vi "mobileye_decoder.vi"(10 "can cluster":T1 {"identifier" format="%03x"}, 11 "name":string="Mobileye560") -> ()   [LabVIEW 2015]
uses:
  rio_Global.vi
panel:
  out "next lane right":dbl[][](array[numeric])
  out "next lane left":dbl[][](array[numeric])
  out "lane_right":dbl[](array[numeric])
  out "lane_left":dbl[](array[numeric])
  out "obs_tmp":dbl[][](array[numeric])
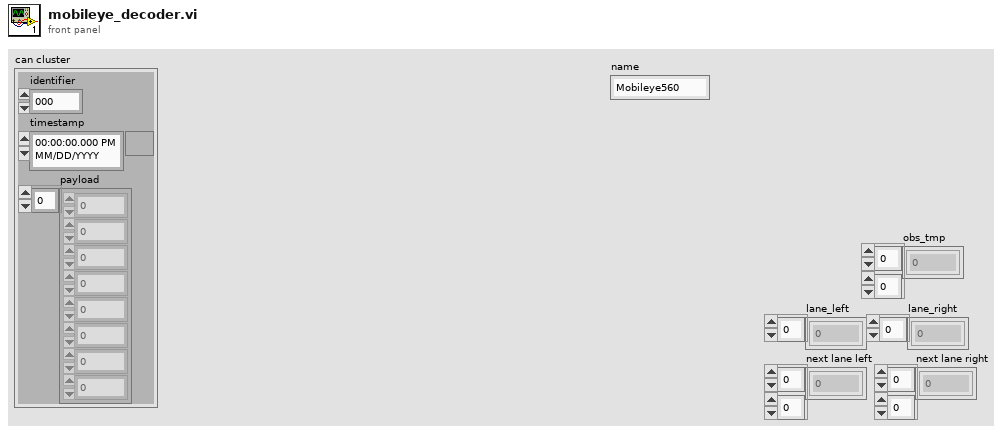
[diagram p1: front panel]
types:
  T1 = cluster{"identifier":u32, "timestamp":timestamp, "payload":u8[]}
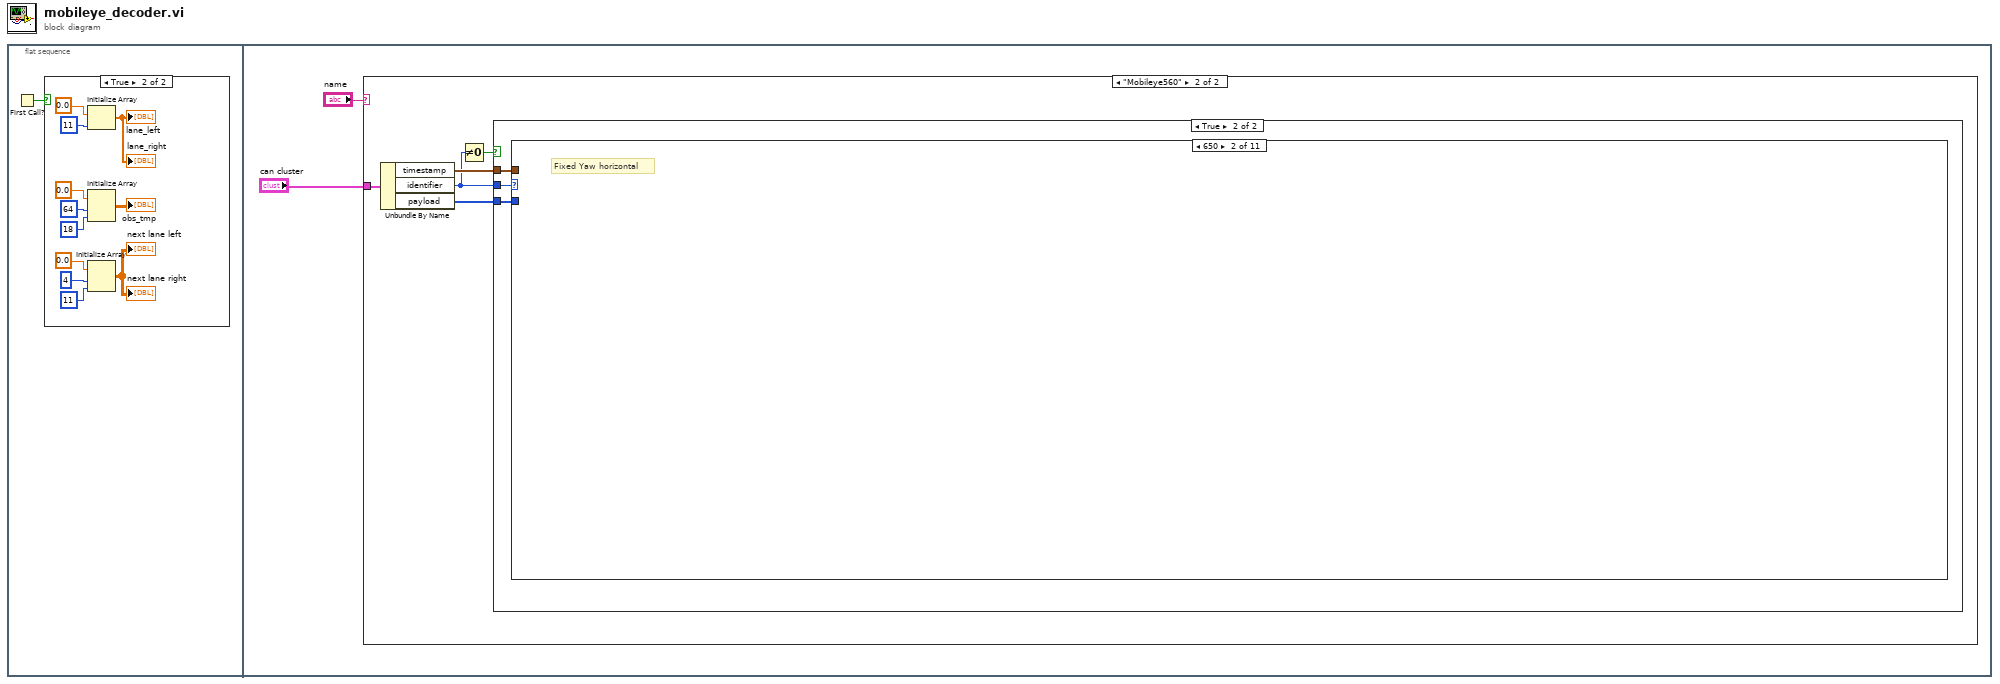
[diagram p0: block diagram]
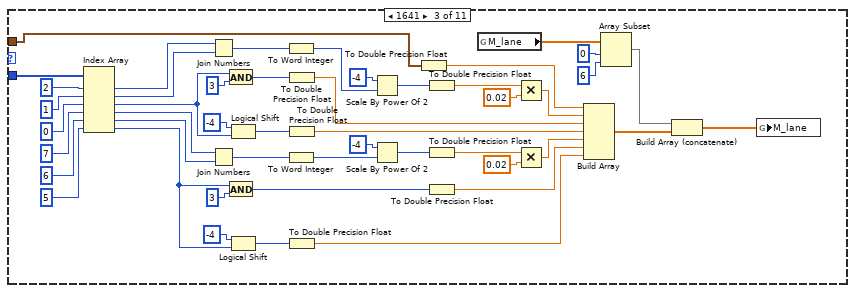
[diagram p6: hidden frame]
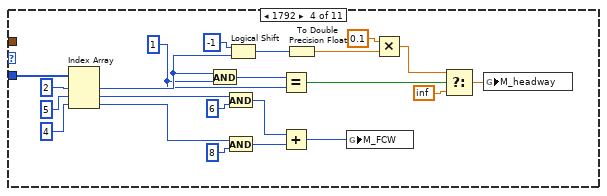
[diagram p7: hidden frame]
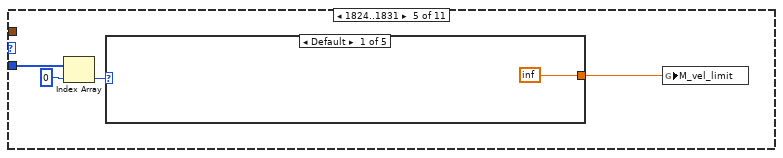
[diagram p8: hidden frame]
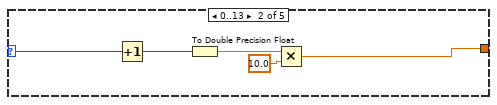
[diagram p9: hidden frame]
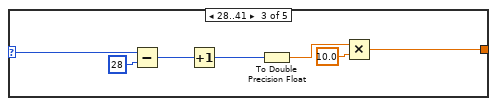
[diagram p10: hidden frame]
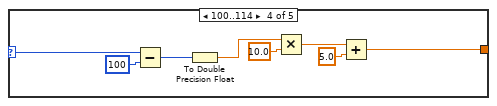
[diagram p11: hidden frame]
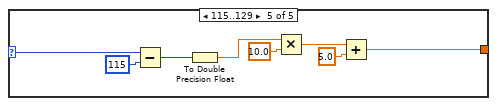
[diagram p12: hidden frame]
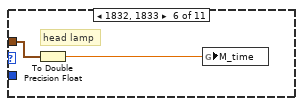
[diagram p13: hidden frame]
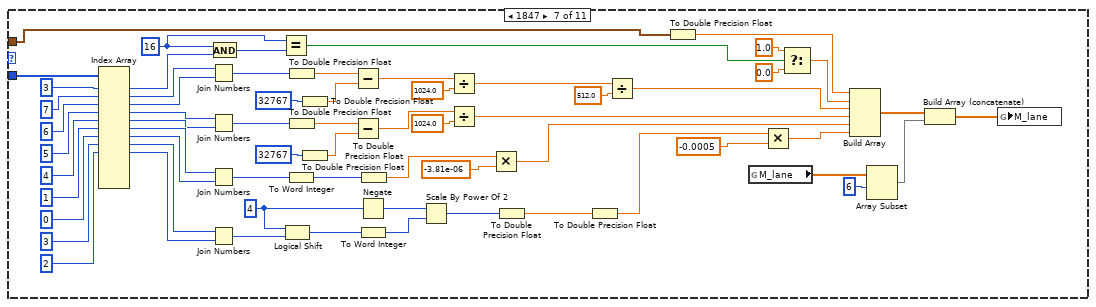
[diagram p14: hidden frame]
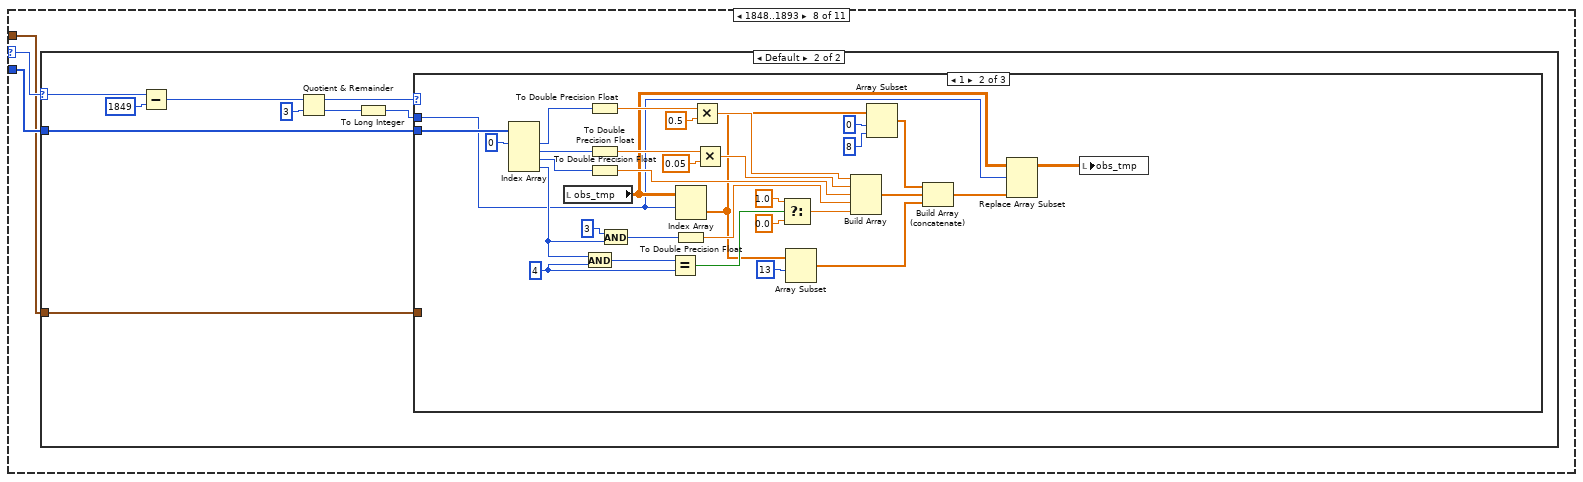
[diagram p15: hidden frame]
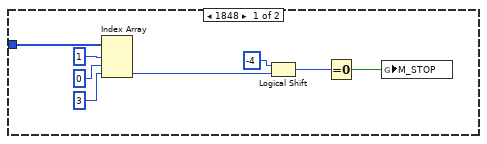
[diagram p16: hidden frame]
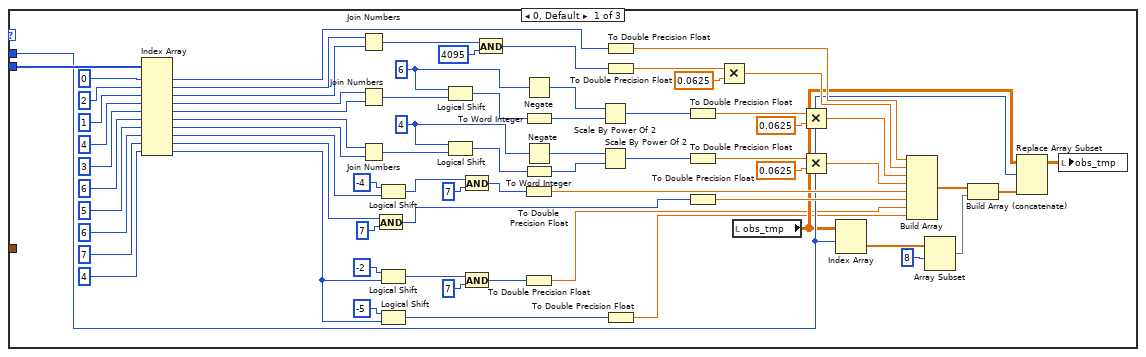
[diagram p17: hidden frame]
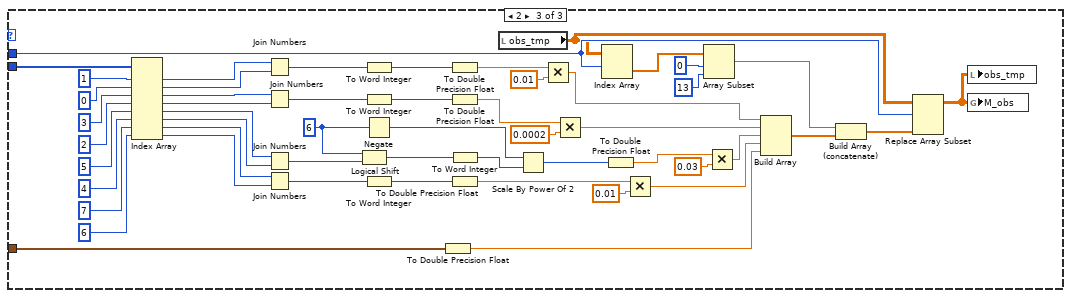
[diagram p18: hidden frame]
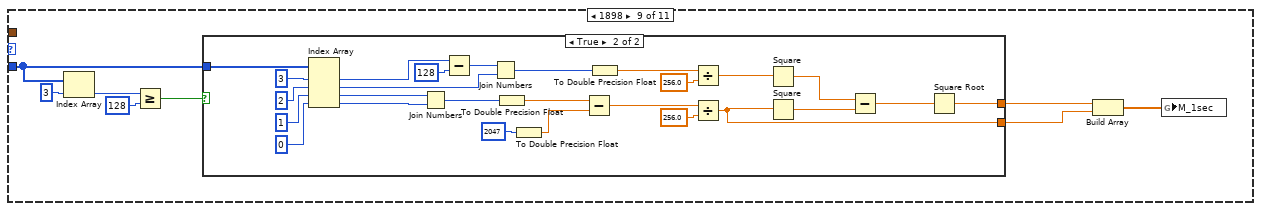
[diagram p19: hidden frame]
diagram:
  n1 = flat-sequence {
    frame #0 {
      n2 = First Call?() -> (First Call?: T/F=w1:bool)
      n3 = case shown="True" w1 {
        frame False {
        }
        frame True {
          n4 = Initialize Array(0.0, 11 ("dimension size")) -> (→"lane_left" →"lane_right":dbl[])
          n5 = Initialize Array(0.0 ("element"), 64 ("dimension size"), 18 ("dimension size")) -> (→"obs_tmp":dbl[][])
          n6 = Initialize Array(0.0, 4 ("dimension size"), 11 ("dimension size")) -> (→"next lane left" →"next lane right":dbl[][])
        }
      }
    }
    frame #1 {
      n7 = case shown="\"Mobileye560\"" "name" {
        tunnel: "can cluster" -> [_ w19]
        frame "False", Default {
        }
        frame "Mobileye560" {
          n8 = Unbundle By Name(w19) -> ("timestamp"=w17:timestamp, "identifier"=w16:u32, "payload"=w18:u8[])
          n9 = Not Equal To 0?(x=w16) -> (x != 0?=w15:bool)
          n10 = case shown="True" w15 {
            tunnel: w18 -> [_ w22]
            tunnel: w17 -> [_ w21]
            tunnel: w16 -> [_ w20]
            frame False {
            }
            frame True {
              n11 = case shown="650" w20 {
                selector: w20 -> [_ _ _ _ _ _ _ w192 _ w399 w480]
                tunnel: w22 -> [_ _ w69 w91 w95 _ w189 w191 w368 w453 w508]
                tunnel: w21 -> [_ _ w46 _ _ w126 w133 w190 _ w419 w483]
                frame 0, Default {
                }
                frame 1616 {
                  # "Fixed Yaw horizontal"
                }
                frame 1641 {
                  n12 = Index Array(array=w69, index #1=2 ("index"), index #2=1 ("index"), index #3=0 ("index"), index #4=7 ("index"), index #5=6 ("index"), index #6=5 ("index")) -> (element #1=w66:u8, element #2=w65:u8, element #3=w44:u8, element #4=w37:u8, element #5=w36:u8, element #6=w32:u8)
                  n13 = Join Numbers(hi=w66, lo=w65) -> ((hi.lo)=w64:u16)
                  n14 = Join Numbers(hi=w37, lo=w36) -> ((hi.lo)=w59:u16)
                  n15 = And(x=w44, y=u8 3) -> (x .and. y?=w43:u8)
                  n16 = And(x=w32, y=u8 3) -> (x .and. y?=w35:u8)
                  n17 = Logical Shift(y=i16 -4, x=w44) -> (x << y=w42:u8)
                  n18 = Logical Shift(y=i16 -4, x=w32) -> (x << y=w39:u8)
                  n19 = To Word Integer(number=w64) -> (16bit integer=w51:i16)
                  n20 = To Word Integer(number=w59) -> (16bit integer=w48:i16)
                  n21 = To Double Precision Float(number=w43) -> (double precision float=w41:dbl)
                  n22 = To Double Precision Float(number=w42) -> (double precision float=w40:dbl)
                  n23 = To Double Precision Float(number=w39) -> (double precision float=w33:dbl)
                  n24 = Scale By Power Of 2(n=i16 -4 ("y"), x=w51) -> (x*2^n=w50:i16)
                  n25 = Scale By Power Of 2(n=i16 -4 ("y"), x=w48) -> (x*2^n=w47:i16)
                  n26 = To Double Precision Float(number=w46) -> (double precision float=w31:dbl)
                  n27 = To Double Precision Float(number=w50) -> (double precision float=w63:dbl)
                  n28 = To Double Precision Float(number=w47) -> (double precision float=w60:dbl)
                  n29 = To Double Precision Float(number=w35) -> (double precision float=w34:dbl)
                  n30 = global read "rio_Global.vi" "M_lane"() -> (w23:dbl[])
                  n31 = Multiply(x=w63, y=0.02) -> (x*y=w26:dbl)
                  n32 = Multiply(x=w60, y=0.02) -> (x*y=w25:dbl)
                  n33 = Build Array(w31, w26, w41, w40, w25, w34, w33) -> (w27:dbl[])
                  n34 = Array Subset(array=w23, index=0, length=6) -> (w28:dbl[])
                  n35 = Build Array (concatenate)(w28, w27) -> (w24:dbl[])
                  n36 = global write "rio_Global.vi" "M_lane"(w24) -> ()
                }
                frame 1792 {
                  w86 = u8 1 ("y")
                  n37 = Index Array(array=w91, index #1=2 ("index"), index #2=5 ("index"), index #3=4 ("index")) -> (element #1=w89:u8, element #2=w78:u8, element #3=w74:u8)
                  n38 = And(x=w89, y=w86) -> (x .and. y?=w87:u8)
                  n39 = And(x=w78, y=u8 6) -> (x .and. y?=w73:u8)
                  n40 = And(x=w74, y=u8 8) -> (x .and. y?=w72:u8)
                  n41 = Logical Shift(y=i16 -1, x=w89) -> (x << y=w84:u8)
                  n42 = Equal?(x=w87, y=w86) -> (x = y?=w85:bool)
                  n43 = Add(x=w73, y=w72) -> (x+y=w70:u8)
                  n44 = To Double Precision Float(number=w84) -> (double precision float=w83:dbl)
                  n45 = global write "rio_Global.vi" "M_FCW"(w70) -> ()
                  n46 = Multiply(x=0.1, y=w83) -> (x*y=w81:dbl)
                  n47 = Select(t=w81, s=w85, f=inf) -> (s? t:f=w71:dbl)
                  n48 = global write "rio_Global.vi" "M_headway"(w71) -> ()
                }
                frame 1824..1831 {
                  n49 = Index Array(array=w95, index=0) -> (element=w93:u8)
                  n50 = case shown="Default" w93 {
                    selector: w93 -> [_ w101 w104 w114 w122]
                    tunnel: [inf w97 w105 w109 w117] -> w92
                    frame Default {
                    }
                    frame 0..13 {
                      n51 = Increment(x=w101) -> (x+1=w100:u8)
                      n52 = To Double Precision Float(number=w100) -> (double precision float=w99:dbl)
                      n53 = Multiply(x=w99, y=10.0) -> (x*y=w97:dbl)
                    }
                    frame 28..41 {
                      n54 = Subtract(x=w104, y=u8 28) -> (x-y=w103:u8)
                      n55 = Increment(x=w103) -> (x+1=w108:u8)
                      n56 = To Double Precision Float(number=w108) -> (double precision float=w107:dbl)
                      n57 = Multiply(x=w107, y=10.0) -> (x*y=w105:dbl)
                    }
                    frame 100..114 {
                      n58 = Subtract(x=w114, y=u8 100) -> (x-y=w112:u8)
                      n59 = To Double Precision Float(number=w112) -> (double precision float=w116:dbl)
                      n60 = Multiply(x=w116, y=10.0) -> (x*y=w111:dbl)
                      n61 = Add(x=w111, y=5.0) -> (x+y=w109:dbl)
                    }
                    frame 115..129 {
                      n62 = Subtract(x=w122, y=u8 115) -> (x-y=w120:u8)
                      n63 = To Double Precision Float(number=w120) -> (double precision float=w124:dbl)
                      n64 = Multiply(x=w124, y=10.0) -> (x*y=w119:dbl)
                      n65 = Add(x=w119, y=5.0) -> (x+y=w117:dbl)
                    }
                  }
                  n66 = global write "rio_Global.vi" "M_vel_limit"(w92) -> ()
                }
                frame 1832, 1833 {
                  # "head lamp"
                  n67 = To Double Precision Float(number=w126) -> (double precision float=w125:dbl)
                  n68 = global write "rio_Global.vi" "M_time"(w125) -> ()
                }
                frame 1847 {
                  w166 = u8 16 ("x")
                  w168 = i16 4 ("x")
                  n69 = Index Array(array=w189, index #1=3 ("index"), index #2=7 ("index"), index #3=6 ("index"), index #4=5 ("index"), index #5=4 ("index"), index #6=1 ("index"), index #7=0 ("index"), index #8=3 ("index"), index #9=2 ("index")) -> (element #1=w149:u8, element #2=w143:u8, element #3=w142:u8, element #4=w141:u8, element #5=w140:u8, element #6=w186:u8, element #7=w185:u8, element #8=w178:u8, element #9=w177:u8)  [unwired: 4 in, 4 out]
                  n70 = Join Numbers(hi=w143, lo=w142) -> ((hi.lo)=w165:u16)
                  n71 = Join Numbers(hi=w141, lo=w140) -> ((hi.lo)=w153:u16)
                  n72 = Join Numbers(hi=w186, lo=w185) -> ((hi.lo)=w184:u16)
                  n73 = Join Numbers(hi=w178, lo=w177) -> ((hi.lo)=w172:u16)
                  n74 = And(x=w166, y=w149) -> (x .and. y?=w167:u8)
                  n75 = Equal?(x=w166, y=w167) -> (x = y?=w152:bool)
                  n76 = Logical Shift(y=w168, x=w172) -> (x << y=w176:u16)
                  n77 = To Word Integer(number=w184) -> (16bit integer=w183:i16)
                  n78 = To Double Precision Float(number=w165) -> (double precision float=w164:dbl)
                  n79 = To Double Precision Float(number=w153) -> (double precision float=w154:dbl)
                  n80 = To Double Precision Float(number=i16 32767) -> (double precision float=w162:dbl)
                  n81 = To Double Precision Float(number=i16 32767) -> (double precision float=w156:dbl)
                  n82 = Subtract(x=w164, y=w162) -> (x-y=w161:dbl)
                  n83 = Subtract(x=w154, y=w156) -> (x-y=w157:dbl)
                  n84 = Negate(x=w168) -> (-x=w171:i16)
                  n85 = To Word Integer(number=w176) -> (16bit integer=w170:i16)
                  n86 = To Double Precision Float(number=w183) -> (double precision float=w182:dbl)
                  n87 = Scale By Power Of 2(n=w171, x=w170) -> (x*2^n=w169:i16)
                  n88 = Divide(x=w161, y=1024.0) -> (x/y=w138:dbl)
                  n89 = Divide(x=w157, y=1024.0) -> (x/y=w136:dbl)
                  n90 = Multiply(x=w182, y=-3.81e-06) -> (x*y=w135:dbl)
                  n91 = To Double Precision Float(number=w169) -> (double precision float=w173:dbl)
                  n92 = To Double Precision Float(number=w173) -> (double precision float=w174:dbl)
                  n93 = Divide(x=w138, y=512.0) -> (x/y=w137:dbl)
                  n94 = To Double Precision Float(number=w133) -> (double precision float=w129:dbl)
                  n95 = global read "rio_Global.vi" "M_lane"() -> (w127:dbl[])
                  n96 = Multiply(x=w174, y=-0.0005) -> (x*y=w134:dbl)
                  n97 = Select(t=1.0, s=w152, f=0.0) -> (s? t:f=w139:dbl)
                  n98 = Build Array(w129, w139, w137, w136, w135, w134) -> (w131:dbl[])
                  n99 = Array Subset(array=w127, index=6) -> (w130:dbl[])  [unwired: 1 in]
                  n100 = Build Array (concatenate)(w131, w130) -> (w128:dbl[])
                  n101 = global write "rio_Global.vi" "M_lane"(w128) -> ()
                }
                frame 1848..1893 {
                  n102 = case shown="Default" w192 {
                    selector: w192 -> [_ w205]
                    tunnel: w191 -> [w200 w204]
                    tunnel: w190 -> [_ w201]
                    frame 1848 {
                      n103 = Index Array(array=w200, index #1=1 ("index"), index #2=0 ("index"), index #3=3 ("index")) -> (element #3=w195:u8)  [unwired: 2 out]
                      n104 = Logical Shift(y=i16 -4, x=w195) -> (x << y=w197:u8)
                      n105 = Equal To 0?(x=w197) -> (x = 0?=w193:bool)
                      n106 = global write "rio_Global.vi" "M_STOP"(w193) -> ()
                    }
                    frame Default {
                      n107 = Subtract(x=w205, y=u32 1849) -> (x-y=w208:u32)
                      n108 = Quotient & Remainder(x=w208, y=u32 3) -> (x-y*floor(x/y)=w206:u32, floor(x/y)=w203:u32)
                      n109 = To Long Integer(number=w203) -> (32bit integer=w202:i32)
                      n110 = case shown="1" w206 {
                        tunnel: w204 -> [w279 w312 w364]
                        tunnel: w202 -> [w233 w287 w363]
                        tunnel: w201 -> [_ _ w315]
                        frame 0, Default {
                          w222 = i16 4 ("y")
                          w226 = i16 6 ("y")
                          n111 = Index Array(array=w279, index #1=0 ("index"), index #2=2 ("index"), index #3=1 ("index"), index #4=4 ("index"), index #5=3 ("index"), index #6=6 ("index"), index #7=5 ("index"), index #8=6 ("index"), index #9=7 ("index"), index #10=4 ("index")) -> (element #1=w271:u8, element #2=w275:u8, element #3=w274:u8, element #4=w263:u8, element #5=w262:u8, element #6=w250:u8, element #7=w249:u8, element #8=w245:u8, element #9=w238:u8, element #10=w212:u8)
                          n112 = Join Numbers(hi=w275, lo=w274) -> ((hi.lo)=w266:u16)
                          n113 = Join Numbers(hi=w263, lo=w262) -> ((hi.lo)=w261:u16)
                          n114 = Join Numbers(hi=w250, lo=w249) -> ((hi.lo)=w251:u16)
                          n115 = And(x=w238, y=u8 7) -> (x .and. y?=w237:u8)
                          n116 = Logical Shift(y=i16 -4, x=w245) -> (x << y=w244:u8)
                          n117 = Logical Shift(y=i16 -2, x=w212) -> (x << y=w214:u8)
                          n118 = Logical Shift(y=i16 -5, x=w212) -> (x << y=w218:u8)
                          n119 = Logical Shift(y=w226, x=w261) -> (x << y=w260:u16)
                          n120 = Logical Shift(y=w222, x=w251) -> (x << y=w252:u16)
                          n121 = And(x=w244, y=u8 7) -> (x .and. y?=w242:u8)
                          n122 = And(x=w214, y=u8 7) -> (x .and. y?=w216:u8)
                          n123 = And(x=w266, y=u16 4095) -> (x .and. y?=w272:u16)
                          n124 = Negate(x=w226) -> (-x=w227:i16)
                          n125 = To Word Integer(number=w260) -> (16bit integer=w225:i16)
                          n126 = Negate(x=w222) -> (-x=w223:i16)
                          n127 = To Word Integer(number=w252) -> (16bit integer=w221:i16)
                          n128 = To Double Precision Float(number=w242) -> (double precision float=w241:dbl)
                          n129 = To Double Precision Float(number=w216) -> (double precision float=w211:dbl)
                          n130 = Scale By Power Of 2(n=w227, x=w225) -> (x*2^n=w224:i16)
                          n131 = Scale By Power Of 2(n=w223, x=w221) -> (x*2^n=w220:i16)
                          n132 = To Double Precision Float(number=w271) -> (double precision float=w268:dbl)
                          n133 = To Double Precision Float(number=w272) -> (double precision float=w270:dbl)
                          n134 = To Double Precision Float(number=w218) -> (double precision float=w210:dbl)
                          n135 = To Double Precision Float(number=w224) -> (double precision float=w257:dbl)
                          n136 = To Double Precision Float(number=w220) -> (double precision float=w254:dbl)
                          n137 = To Double Precision Float(number=w237) -> (double precision float=w236:dbl)
                          n138 = Multiply(x=w270, y=0.0625) -> (x*y=w267:dbl)
                          n139 = local read "obs_tmp"() -> (w232:dbl[][])
                          n140 = Multiply(x=w257, y=0.0625) -> (x*y=w258:dbl)
                          n141 = Multiply(x=w254, y=0.0625) -> (x*y=w248:dbl)
                          n142 = Index Array(array=w232, index (row)=w233) -> (element=w230:dbl[])  [unwired: 1 in]
                          n143 = Build Array(w268, w267, w258, w248, w241, w236, w211, w210) -> (w235:dbl[])
                          n144 = Array Subset(array=w230, index=8) -> (w229:dbl[])  [unwired: 1 in]
                          n145 = Build Array (concatenate)(w235, w229) -> (w234:dbl[])
                          n146 = Replace Array Subset(array=w232, new element=w234, index (row)=w233) -> (w231:dbl[][])  [unwired: 1 in]
                          n147 = local write "obs_tmp"(w231) -> ()
                        }
                        frame 1 {
                          w297 = u8 4 ("y")
                          n148 = Index Array(array=w312, index #1=0 ("index")) -> (element #1=w310:u8, element #2=w304:u8, element #3=w302:u8, element #4=w291:u8)  [unwired: 3 in]
                          n149 = local read "obs_tmp"() -> (w289:dbl[][])
                          n150 = And(x=w291, y=w297) -> (x .and. y?=w298:u8)
                          n151 = To Double Precision Float(number=w310) -> (double precision float=w309:dbl)
                          n152 = To Double Precision Float(number=w304) -> (double precision float=w305:dbl)
                          n153 = To Double Precision Float(number=w302) -> (double precision float=w301:dbl)
                          n154 = And(x=u8 3 ("y"), y=w291) -> (x .and. y?=w300:u8)
                          n155 = Equal?(x=w298, y=w297) -> (x = y?=w296:bool)
                          n156 = Index Array(array=w289, index (row)=w287) -> (element=w284:dbl[])  [unwired: 1 in]
                          n157 = To Double Precision Float(number=w300) -> (double precision float=w299:dbl)
                          n158 = Multiply(x=w309, y=0.5) -> (x*y=w307:dbl)
                          n159 = Multiply(x=w305, y=0.05) -> (x*y=w303:dbl)
                          n160 = Select(t=1.0, s=w296, f=0.0) -> (s? t:f=w293:dbl)
                          n161 = Array Subset(array=w284, index=13) -> (w280:dbl[])  [unwired: 1 in]
                          n162 = Build Array(w307, w303, w301, w299, w293) -> (w281:dbl[])
                          n163 = Array Subset(array=w284, index=0, length=8) -> (w282:dbl[])
                          n164 = Build Array (concatenate)(w282, w281, w280) -> (w290:dbl[])
                          n165 = Replace Array Subset(array=w289, new element=w290, index (row)=w287) -> (w288:dbl[][])  [unwired: 1 in]
                          n166 = local write "obs_tmp"(w288) -> ()
                        }
                        frame 2 {
                          w337 = i16 6 ("y")
                          n167 = Index Array(array=w364, index #1=1 ("index"), index #2=0 ("index"), index #3=3 ("index"), index #4=2 ("index"), index #5=5 ("index"), index #6=4 ("index"), index #7=7 ("index"), index #8=6 ("index")) -> (element #1=w360:u8, element #2=w359:u8, element #3=w347:u8, element #4=w346:u8, element #5=w342:u8, element #6=w341:u8, element #7=w325:u8, element #8=w324:u8)
                          n168 = Join Numbers(hi=w360, lo=w359) -> ((hi.lo)=w358:u16)
                          n169 = Join Numbers(hi=w347, lo=w346) -> ((hi.lo)=w348:u16)
                          n170 = Join Numbers(hi=w342, lo=w341) -> ((hi.lo)=w340:u16)
                          n171 = Join Numbers(hi=w325, lo=w324) -> ((hi.lo)=w326:u16)
                          n172 = Logical Shift(y=w337, x=w340) -> (x << y=w339:u16)
                          n173 = To Word Integer(number=w358) -> (16bit integer=w357:i16)
                          n174 = To Word Integer(number=w348) -> (16bit integer=w349:i16)
                          n175 = Negate(x=w337) -> (-x=w338:i16)
                          n176 = To Word Integer(number=w326) -> (16bit integer=w327:i16)
                          n177 = To Double Precision Float(number=w315) -> (double precision float=w314:dbl)
                          n178 = To Double Precision Float(number=w357) -> (double precision float=w356:dbl)
                          n179 = To Double Precision Float(number=w349) -> (double precision float=w350:dbl)
                          n180 = To Word Integer(number=w339) -> (16bit integer=w336:i16)
                          n181 = To Double Precision Float(number=w327) -> (double precision float=w328:dbl)
                          n182 = local read "obs_tmp"() -> (w322:dbl[][])
                          n183 = Scale By Power Of 2(n=w338, x=w336) -> (x*2^n=w335:i16)
                          n184 = Multiply(x=w356, y=0.01) -> (x*y=w354:dbl)
                          n185 = Multiply(x=w350, y=0.0002) -> (x*y=w345:dbl)
                          n186 = Index Array(array=w322, index (row)=w363) -> (element=w319:dbl[])  [unwired: 1 in]
                          n187 = To Double Precision Float(number=w335) -> (double precision float=w333:dbl)
                          n188 = Multiply(x=w328, y=0.01) -> (x*y=w323:dbl)
                          n189 = Array Subset(array=w319, index=0, length=13) -> (w316:dbl[])
                          n190 = Multiply(x=w333, y=0.03) -> (x*y=w332:dbl)
                          n191 = Build Array(w354, w345, w332, w323, w314) -> (w318:dbl[])
                          n192 = Build Array (concatenate)(w316, w318) -> (w317:dbl[])
                          n193 = Replace Array Subset(array=w322, new element=w317, index (row)=w363) -> (w313:dbl[][])  [unwired: 1 in]
                          n194 = local write "obs_tmp"(w313) -> ()
                          n195 = global write "rio_Global.vi" "M_obs"(w313) -> ()
                        }
                      }
                    }
                  }
                }
                frame 1898 {
                  n196 = Index Array(array=w368, index=3) -> (element=w371:u8)
                  n197 = Greater Or Equal?(x=w371, y=u8 128) -> (x >= y?=w369:bool)
                  n198 = case shown="True" w369 {
                    tunnel: w368 -> [_ w398]
                    tunnel: [_ w373] -> w367
                    tunnel: [_ w375] -> w366
                    frame False {
                    }
                    frame True {
                      n199 = Index Array(array=w398, index #1=3 ("index"), index #2=2 ("index"), index #3=1 ("index"), index #4=0 ("index")) -> (element #1=w389:u8, element #2=w393:u8, element #3=w392:u8, element #4=w391:u8)
                      n200 = Join Numbers(hi=w392, lo=w391) -> ((hi.lo)=w379:u16)
                      n201 = Subtract(x=w389, y=u8 128) -> (x-y=w388:u8)
                      n202 = Join Numbers(hi=w388, lo=w393) -> ((hi.lo)=w381:u16)
                      n203 = To Double Precision Float(number=w379) -> (double precision float=w387:dbl)
                      n204 = To Double Precision Float(number=u16 2047 ("(hi.lo)")) -> (double precision float=w386:dbl)
                      n205 = Subtract(x=w387, y=w386) -> (x-y=w384:dbl)
                      n206 = To Double Precision Float(number=w381) -> (double precision float=w380:dbl)
                      n207 = Divide(x=w380, y=256.0) -> (x/y=w378:dbl)
                      n208 = Divide(x=w384, y=256.0) -> (x/y=w375:dbl)
                      n209 = Square(x=w378) -> (x^2=w377:dbl)
                      n210 = Square(x=w375) -> (x^2=w376:dbl)
                      n211 = Subtract(x=w377, y=w376) -> (x-y=w374:dbl)
                      n212 = Square Root(x=w374) -> (sqrt(x)=w373:dbl)
                    }
                  }
                  n213 = Build Array(w367, w366) -> (w365:dbl[])
                  n214 = global write "rio_Global.vi" "M_1sec"(w365) -> ()
                }
                frame 1894, 1896, 1900, 1902, 1904, 1906, 1908, 1910, 1912, 1914 {
                  n215 = Index Array(array=w453, index #1=0 ("index"), index #2=7 ("index"), index #3=2 ("index"), index #4=1 ("index"), index #5=4 ("index"), index #6=3 ("index"), index #7=6 ("index"), index #8=5 ("index")) -> (element #1=w409:u8, element #2=w404:u8, element #3=w451:u8, element #4=w450:u8, element #5=w443:u8, element #6=w442:u8, element #7=w433:u8, element #8=w432:u8)
                  n216 = Join Numbers(hi=w451, lo=w450) -> ((hi.lo)=w449:u16)
                  n217 = Join Numbers(hi=w443, lo=w442) -> ((hi.lo)=w441:u16)
                  n218 = Join Numbers(hi=w433, lo=w432) -> ((hi.lo)=w426:u16)
                  n219 = And(x=w409, y=u8 48) -> (x .and. y?=w414:u8)
                  n220 = To Word Integer(number=w449) -> (16bit integer=w448:i16)
                  n221 = To Double Precision Float(number=w441) -> (double precision float=w438:dbl)
                  n222 = To Double Precision Float(number=w426) -> (double precision float=w429:dbl)
                  n223 = Logical Shift(y=i16 -4, x=w414) -> (x << y=w412:u8)
                  n224 = To Double Precision Float(number=u16 32767 ("y")) -> (double precision float=w439:dbl)
                  n225 = To Double Precision Float(number=u16 32767 ("y")) -> (double precision float=w428:dbl)
                  n226 = Logical Shift(y=28, x=1) -> (x << y=w423:i32)
                  n227 = Subtract(x=w438, y=w439) -> (x-y=w437:dbl)
                  n228 = Subtract(x=w429, y=w428) -> (x-y=w421:dbl)
                  n229 = To Double Precision Float(number=w423) -> (double precision float=w422:dbl)
                  n230 = Logical Shift(y=i16 -6, x=w409) -> (x << y=w407:u8)
                  n231 = Divide(x=w448, y=i16 256) -> (x/y=w434:dbl)
                  n232 = Divide(x=w421, y=w422) -> (x/y=w420:dbl)
                  n233 = To Double Precision Float(number=w412) -> (double precision float=w410:dbl)
                  n234 = And(x=u8 15, y=w409) -> (x .and. y?=w416:u8)
                  n235 = Multiply(x=w404, y=0.01) -> (x*y=w402:dbl)
                  n236 = To Double Precision Float(number=w419) -> (double precision float=w401:dbl)
                  n237 = Divide(x=w437, y=1024000.0) -> (x/y=w435:dbl)
                  n238 = To Double Precision Float(number=w416) -> (double precision float=w411:dbl)
                  n239 = To Double Precision Float(number=w407) -> (double precision float=w406:dbl)
                  n240 = Build Array(w401, w411, w410, w406, w402, w434, w435, w420) -> (w400:dbl[])
                  n241 = case shown="766" w399 {
                    selector: w399 -> [_ _ _ w469 w477]
                    tunnel: w400 -> [_ w455 w461 w470 w478]
                    frame 0, Default {
                    }
                    frame 1894 {
                      n242 = local read "lane_left"() -> (w458:dbl[])
                      n243 = Array Subset(array=w458, index=8) -> (w456:dbl[])  [unwired: 1 in]
                      n244 = Build Array (concatenate)(w455, w456) -> (w454:dbl[])
                      n245 = local write "lane_left"(w454) -> ()
                    }
                    frame 1896 {
                      n246 = local read "lane_right"() -> (w463:dbl[])
                      n247 = Array Subset(array=w463, index=8) -> (w460:dbl[])  [unwired: 1 in]
                      n248 = Build Array (concatenate)(w461, w460) -> (w459:dbl[])
                      n249 = local write "lane_right"(w459) -> ()
                    }
                    frame 1900, 1904, 1908, 1912 {
                      n250 = Subtract(x=w469, y=u32 1900) -> (x-y=w467:u32)
                      n251 = Quotient & Remainder(x=w467, y=u32 4) -> (floor(x/y)=w465:u32)  [unwired: 1 out]
                      n252 = local read "next lane left"() -> (w471:dbl[][])
                      n253 = Replace Array Subset(array=w471, new element=w470, index (row)=w465) -> (w464:dbl[][])  [unwired: 1 in]
                      n254 = local write "next lane left"(w464) -> ()
                    }
                    frame 1902, 1906, 1910, 1914 {
                      n255 = Subtract(x=w477, y=u32 1900) -> (x-y=w475:u32)
                      n256 = Quotient & Remainder(x=w475, y=u32 4) -> (floor(x/y)=w473:u32)  [unwired: 1 out]
                      n257 = local read "next lane right"() -> (w479:dbl[][])
                      n258 = Replace Array Subset(array=w479, new element=w478, index (row)=w473) -> (w472:dbl[][])  [unwired: 1 in]
                      n259 = local write "next lane right"(w472) -> ()
                    }
                  }
                }
                frame 1895, 1897, 1901, 1903, 1905, 1907, 1909, 1911, 1913, 1915 {
                  w490 = u16 32768 ("y")
                  n260 = Index Array(array=w508, index #1=1 ("index"), index #2=0 ("index"), index #3=3 ("index"), index #4=2 ("index")) -> (element #1=w505:u8, element #2=w504:u8, element #3=w495:u8, element #4=w494:u8)
                  n261 = Join Numbers(hi=w505, lo=w504) -> ((hi.lo)=w500:u16)
                  n262 = Join Numbers(hi=w495, lo=w494) -> ((hi.lo)=w491:u16)
                  n263 = Subtract(x=w491, y=w490) -> (x-y=w489:u16)
                  n264 = And(x=w490, y=w491) -> (x .and. y?=w493:u16)
                  n265 = To Double Precision Float(number=w500) -> (double precision float=w501:dbl)
                  n266 = To Double Precision Float(number=u16 32767 ("y")) -> (double precision float=w502:dbl)
                  n267 = Subtract(x=w501, y=w502) -> (x-y=w499:dbl)
                  n268 = Equal?(x=w490, y=w493) -> (x = y?=w492:bool)
                  n269 = Divide(x=w489, y=u16 256) -> (x/y=w487:dbl)
                  n270 = Select(t=w487, s=w492, f=0.0) -> (s? t:f=w484:dbl)
                  n271 = Divide(x=w499, y=1024.0) -> (x/y=w485:dbl)
                  n272 = To Double Precision Float(number=w483) -> (double precision float=w482:dbl)
                  n273 = Build Array(w482, w485, w484) -> (w481:dbl[])
                  n274 = case shown="76F, 773, 777, 77B" w480 {
                    selector: w480 -> [_ _ _ w530 w545]
                    tunnel: w481 -> [_ w510 w516 w526 w541]
                    frame 0, Default {
                    }
                    frame 1895 {
                      n275 = local read "lane_left"() -> (w514:dbl[])
                      n276 = Array Subset(array=w514, index=0, length=8 ("index")) -> (w513:dbl[])
                      n277 = Build Array (concatenate)(w513, w510) -> (w509:dbl[])
                      n278 = local write "lane_left"(w509) -> ()
                      n279 = global write "rio_Global.vi" "M_lane_left"(w509) -> ()
                    }
                    frame 1897 {
                      n280 = local read "lane_right"() -> (w520:dbl[])
                      n281 = Array Subset(array=w520, index=0, length=8 ("index")) -> (w519:dbl[])
                      n282 = Build Array (concatenate)(w519, w516) -> (w515:dbl[])
                      n283 = local write "lane_right"(w515) -> ()
                      n284 = global write "rio_Global.vi" "M_lane_right"(w515) -> ()
                    }
                    frame 1901, 1905, 1909, 1913 {
                      n285 = Subtract(x=w530, y=u32 1900) -> (x-y=w533:u32)
                      n286 = local read "next lane left"() -> (w535:dbl[][])
                      n287 = Quotient & Remainder(x=w533, y=u32 4) -> (floor(x/y)=w527:u32)  [unwired: 1 out]
                      n288 = Index Array(array=w526, index #1=0 ("index")) -> (element #1=w524:dbl, element #2=w523:dbl, element #3=w522:dbl)  [unwired: 2 in]
                      n289 = Replace Array Subset(array=w535, new element #1=w524, index (row) #1=w527, index (col) #1=8 ("disabled index (col)"), new element #2=w523, index (row) #2=w527, index (col) #2=9 ("disabled index (col)"), new element #3=w522, index (row) #3=w527, index (col) #3=10 ("index (col)")) -> (w521:dbl[][])
                      n290 = local write "next lane left"(w521) -> ()
                      n291 = global write "rio_Global.vi" "M_next lane left"(w521) -> ()
                    }
                    frame 1903, 1907, 1911, 1915 {
                      n292 = Subtract(x=w545, y=u32 1900) -> (x-y=w548:u32)
                      n293 = local read "next lane right"() -> (w550:dbl[][])
                      n294 = Quotient & Remainder(x=w548, y=u32 4) -> (floor(x/y)=w542:u32)  [unwired: 1 out]
                      n295 = Index Array(array=w541, index #1=0 ("index")) -> (element #1=w539:dbl, element #2=w538:dbl, element #3=w537:dbl)  [unwired: 2 in]
                      n296 = Replace Array Subset(array=w550, new element #1=w539, index (row) #1=w542, index (col) #1=8 ("disabled index (col)"), new element #2=w538, index (row) #2=w542, index (col) #2=9 ("disabled index (col)"), new element #3=w537, index (row) #3=w542, index (col) #3=10 ("index (col)")) -> (w536:dbl[][])
                      n297 = local write "next lane right"(w536) -> ()
                      n298 = global write "rio_Global.vi" "M_next lane right"(w536) -> ()
                    }
                  }
                }
              }
            }
          }
        }
      }
    }
  }
